vi "test pass.vi"(8 "error in (no error)":errorcluster, 11 "Passing test in":refnum<class "LUnit test 2.lvclass">) -> (0 "error out":errorcluster, 3 "Passing test out":refnum<class "LUnit test 2.lvclass">)   [LabVIEW 2020, in "LUnit test 2.lvclass"]
uses:
  LUnit test 2.lvclass
  C:/Program Files (x86)/National Instruments/LabVIEW 2020/vi.lib/Asteme/LUnit/Test Case.lvclass
  <vilib>/Asteme/LUnit/Test Case.lvclass/Test Case.ctl
  <vilib>/Asteme/LUnit/LUnit Assertion Result.lvclass/LUnit Assertion Result.ctl
  <vilib>/Asteme/LUnit/LUnit Test Case Result.lvclass/LUnit Test Case Result.ctl
  <vilib>/Asteme/LUnit/LUnit Method Result.lvclass/LUnit Method Result.ctl
  <vilib>/Asteme/LUnit/Palette/Fail.vi
  <vilib>/Asteme/LUnit/Palette/Pass.vi
  <vilib>/Asteme/LUnit/Set Assertion Type.vi
  <vilib>/Asteme/LUnit/Add test result.vi
  <vilib>/Asteme/LUnit/LUnit Write Passed.vi
  <vilib>/Asteme/LUnit/LUnit Write Message.vi
  <vilib>/Asteme/LUnit/LUnit Write Description.vi
  <vilib>/Asteme/LUnit/LUnit Write Assertion Type.vi
  <vilib>/Asteme/LUnit/LUnit Record Assertion Result.vi
  <vilib>/Asteme/LUnit/LUnit Aggregate Assertion Results.vi
  <vilib>/Asteme/LUnit/Assertion Result/LUnit Read Status.vi
  <vilib>/Asteme/LUnit/LUnit Read Message.vi
  <vilib>/Asteme/LUnit/LUnit Read Description.vi
  <vilib>/Asteme/LUnit/Method Result/LUnit Merge Status.vi
  <vilib>/Asteme/LUnit/LUnit Concatenate result strings.vi
  <vilib>/Asteme/LUnit/LUnit Assertion Result.lvclass
  <vilib>/Asteme/LUnit/Test Case.lvclass
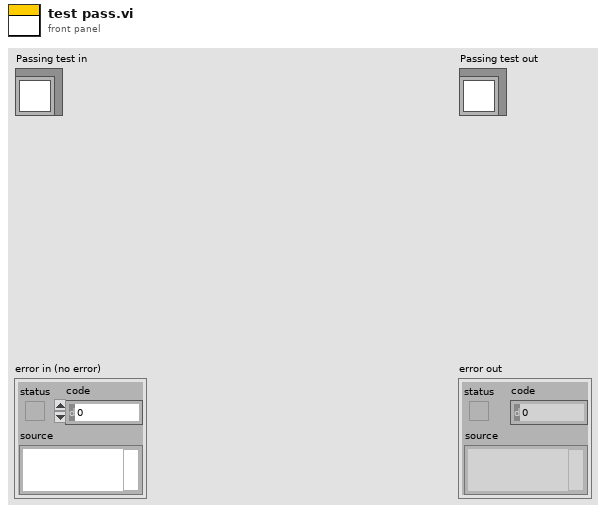
[diagram p1: front panel]
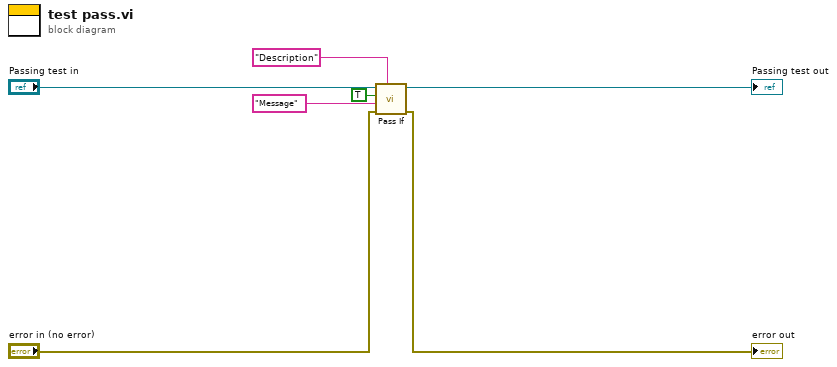
[diagram p0: block diagram]
diagram:
  n1 = call <vilib>:"Pass If.vi"("Description"="Description", "error in (no error)"="error in (no error)", "Message"="Message", "Pass?"=TRUE, "LUnit Test Case In"="Passing test in") -> ("error out"=→"error out":errorcluster, "LUnit Test Case Out"=→"Passing test out":refnum<class "LUnit test 2.lvclass">)  [unwired: 5 in]
